vi "Actuators Move Absolute.vi"(0 "Notifier Name":string, 2 "Wait to Finish":bool, 5 "Channel":i32[](array[numeric]), 7 "Position":dbl[](array[numeric]), 11 "Error In":errorcluster) -> (4 "Notifier Name Out":string, 15 "Error Out":errorcluster)   [LabVIEW 2020]
uses:
  Actuators Controls/Actuators Note Type.ctl
  Actuators Controls/Actuators Actions.ctl
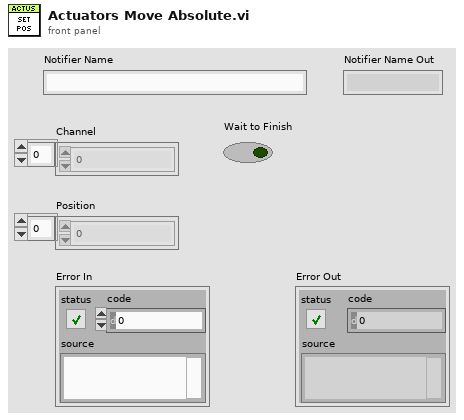
[diagram p1: front panel]
types:
  T1 = typedef "Actuators Note Type.ctl" = cluster{"Actions":T2, "Cmd Received ":bool, "Setpoint":dbl[], "Position":dbl[], "Channel":i32[], "Jog Step":dbl[], "Velocity":dbl[], "Acceleration":dbl[]}
  T2 = typedef "Actuators Actions.ctl" = enum16{"Nothing", "Get Position", "Get Acceleration", "Get Velocity", "Get Jog Step", "Set Acceleration", "Set Velocity", "Set Jog Step", "Move Absolute", "Move Relative", "Jog Forward", "Jog Reverse", "Halt", "Quit"}
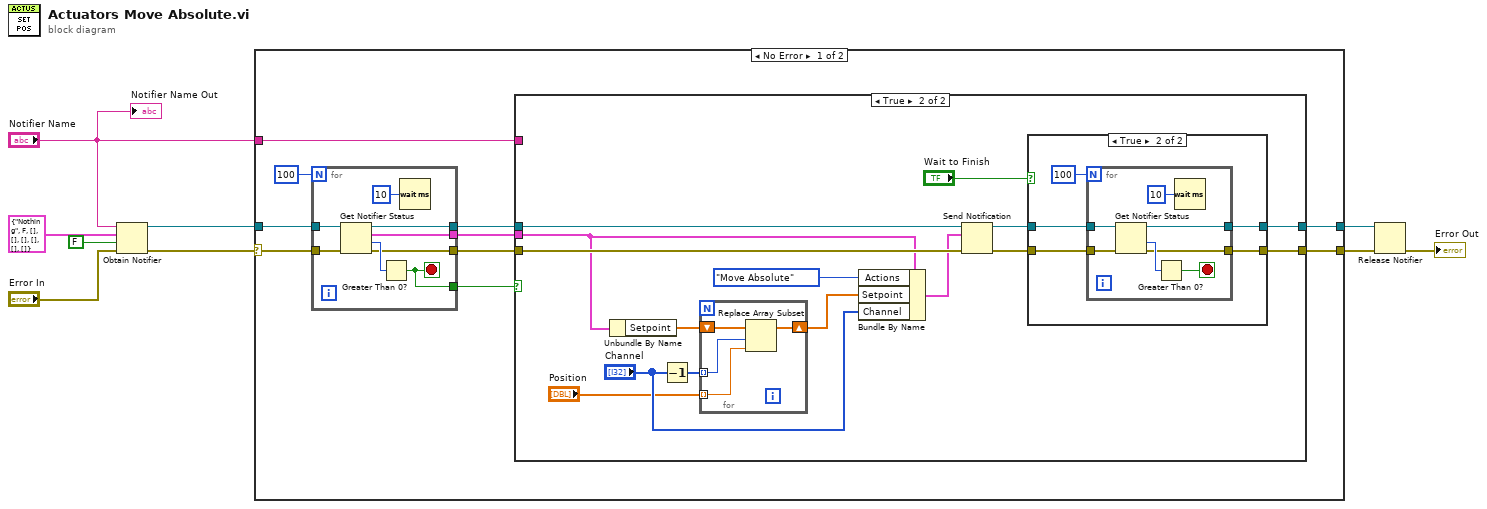
[diagram p0: block diagram]
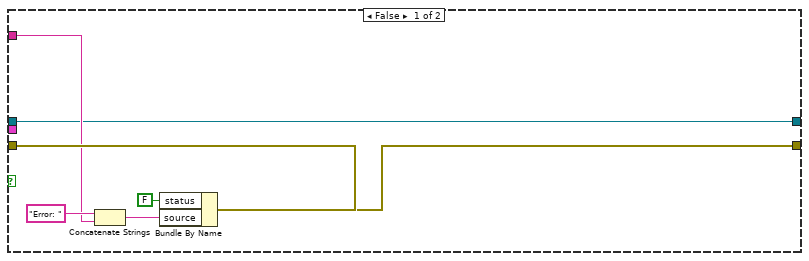
[diagram p2: hidden frame]
diagram:
  n1 = Obtain Notifier(name (unnamed)="Notifier Name", notification data type=T1 {"Actions"=enum."Nothing", "Cmd Received "=FALSE, "Setpoint"=[], "Position"=[], "Channel"=[], "Jog Step"=[], "Velocity"=[], "Acceleration"=[]} ("Actuators Note"), create if not found? (T)=FALSE, error in (no error)="Error In") -> (notifier out=w5:refnum<notifier>, error out=w8:errorcluster)  [unwired: 1 out]
  n2 = case shown="No Error" w8 {
    selector: w8 -> [w17 w68]
    tunnel: w5 -> [w18 w69]
    tunnel: "Notifier Name" -> [w12 _]
    tunnel: [w11 w69] -> w4
    tunnel: [w10 w68] -> w3
    frame No Error {
      n3 = for {
        N: 100 -> [_]
        tunnel: [w66] -> w14
        tunnel: w18 -> [w67]
        tunnel: [w65] -> w15
        tunnel: w17 -> [w62]
        tunnel: [w61] -> w16
        tunnel: [w60] -> w13
        stop <- w61 stop-if-true
        n4 = Get Notifier Status(notifier=w67, error in (no error)=w62) -> (notifier out=w65:refnum<notifier>, current notification=w66:T1, # waiting=w64:i32, error out=w60:errorcluster)  [unwired: 1 out]
        n5 = Greater Than 0?(x=w64) -> (x > 0?=w61:bool)
        n6 = Wait (ms)(milliseconds to wait=u32 10) -> ()  [unwired: 1 out]
      }
      n7 = case shown="True" w16 {
        tunnel: w15 -> [w21 w41]
        tunnel: w14 -> [_ w29]
        tunnel: w13 -> [w26 w40]
        tunnel: w12 -> [w22 _]
        tunnel: [w21 w36] -> w11
        tunnel: [w20 w37] -> w10
        frame False {
          n8 = Concatenate Strings("Error: " ("source"), w22) -> (w23:string)
          n9 = Bundle By Name(cluster=w26, "status"=FALSE, "source"=w23) -> (w20:errorcluster)
        }
        frame True {
          n10 = Unbundle By Name(w29) -> ("Setpoint"=w34:dbl[])
          n11 = Decrement(x="Channel") -> (x-1=w32:i32[])
          n12 = for {
            tunnel: w32 -> [w45] mode=indexing
            tunnel: "Position" -> [w44] mode=indexing
            shift-right: [w42] -> w33
            shift-left: w34 -> [w43]
            n13 = Replace Array Subset(array=w43, new element=w44, index=w45) -> (w42:dbl[])
          }
          n14 = Bundle By Name(cluster=w29, "Actions"=Actuators_Actions."Move Absolute", "Setpoint"=w33, "Channel"="Channel") -> (w30:T1)
          n15 = Send Notification(notification=w30, notifier=w41, error in (no error)=w40) -> (notifier out=w39:refnum<notifier>, error out=w38:errorcluster)
          n16 = case shown="True" "Wait to Finish" {
            tunnel: w39 -> [w47 w51]
            tunnel: w38 -> [w46 w50]
            tunnel: [w46 w49] -> w37
            tunnel: [w47 w48] -> w36
            frame False {
            }
            frame True {
              n17 = for {
                N: 100 -> [_]
                tunnel: w51 -> [w59]
                tunnel: [w58] -> w48
                tunnel: w50 -> [w55]
                tunnel: [w53] -> w49
                stop <- w54 stop-if-true
                n18 = Get Notifier Status(notifier=w59, error in (no error)=w55) -> (notifier out=w58:refnum<notifier>, # waiting=w57:i32, error out=w53:errorcluster)  [unwired: 2 out]
                n19 = Greater Than 0?(x=w57) -> (x > 0?=w54:bool)
                n20 = Wait (ms)(milliseconds to wait=u32 10) -> ()  [unwired: 1 out]
              }
            }
          }
        }
      }
    }
    frame Error {
    }
  }
  n21 = Release Notifier(notifier=w4, error in (no error)=w3) -> (error out=→"Error Out":errorcluster)  [unwired: 1 in, 2 out]
  "Notifier Name Out" <- "Notifier Name"
